vi "PI Controller with Stability Checker and Rate Limiter.vi"(2 "PI Parameters":T2, 3 "Tolerances":dbl[](array[numeric]), 4 "Feedback":dbl[](array[numeric]), 5 "CtrlIndex":i32, 7 "CommandCluster":T4, 9 "CmdLimits":cluster{"Step":dbl, "Max":dbl, "Min":dbl}, 10 "Rate Limits":T1={"Distant Rate"=50.0, "Close Rate"=0.5, "Error Cutoff"=10.0}, 11 "Stability In":T3, 12 "Controller?":bool, 13 "FF Scales":dbl[][](array[numeric])=[[0.0, 0.0, 0.0]]) -> (6 "Output":dbl, 8 "PIdata":dbl[](array[numeric]), 14 "Stable?":bool, 15 "Stability Out":T3)   [LabVIEW 2013]
uses:
  TypeDef/Command Cluster.ctl
  TypeDef/PI Parameters.ctl
  <vilib>/addons/control/pid/pid.llb/PID Output Rate Limiter (DBL).vi
  <vilib>/addons/control/pid/NI_PID_pid.lvlib
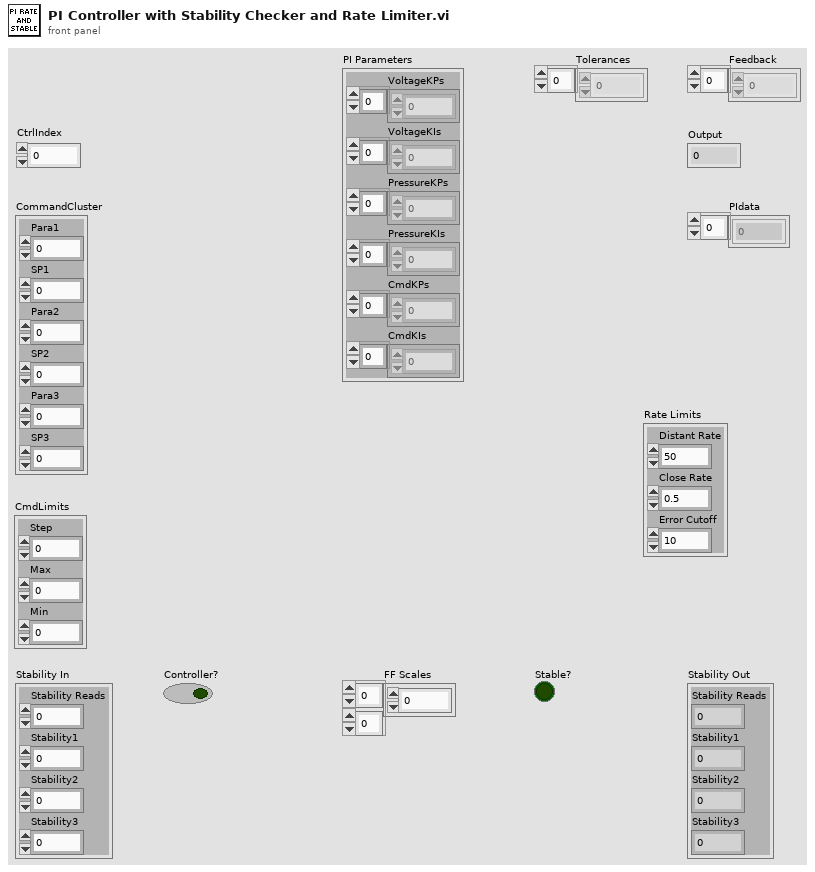
[diagram p1: front panel]
types:
  T1 = cluster{"Distant Rate":dbl, "Close Rate":dbl, "Error Cutoff":dbl}
  T2 = typedef "PI Parameters.ctl" = cluster{"VoltageKPs":dbl[], "VoltageKIs":dbl[], "PressureKPs":dbl[], "PressureKIs":dbl[], "CmdKPs":dbl[], "CmdKIs":dbl[]}
  T3 = cluster{"Stability Reads":i32, "Stability1":i32, "Stability2":i32, "Stability3":i32}
  T4 = typedef "Command Cluster.ctl" = cluster{"Para1":i32, "SP1":dbl, "Para2":i32, "SP2":dbl, "Para3":i32, "SP3":dbl}
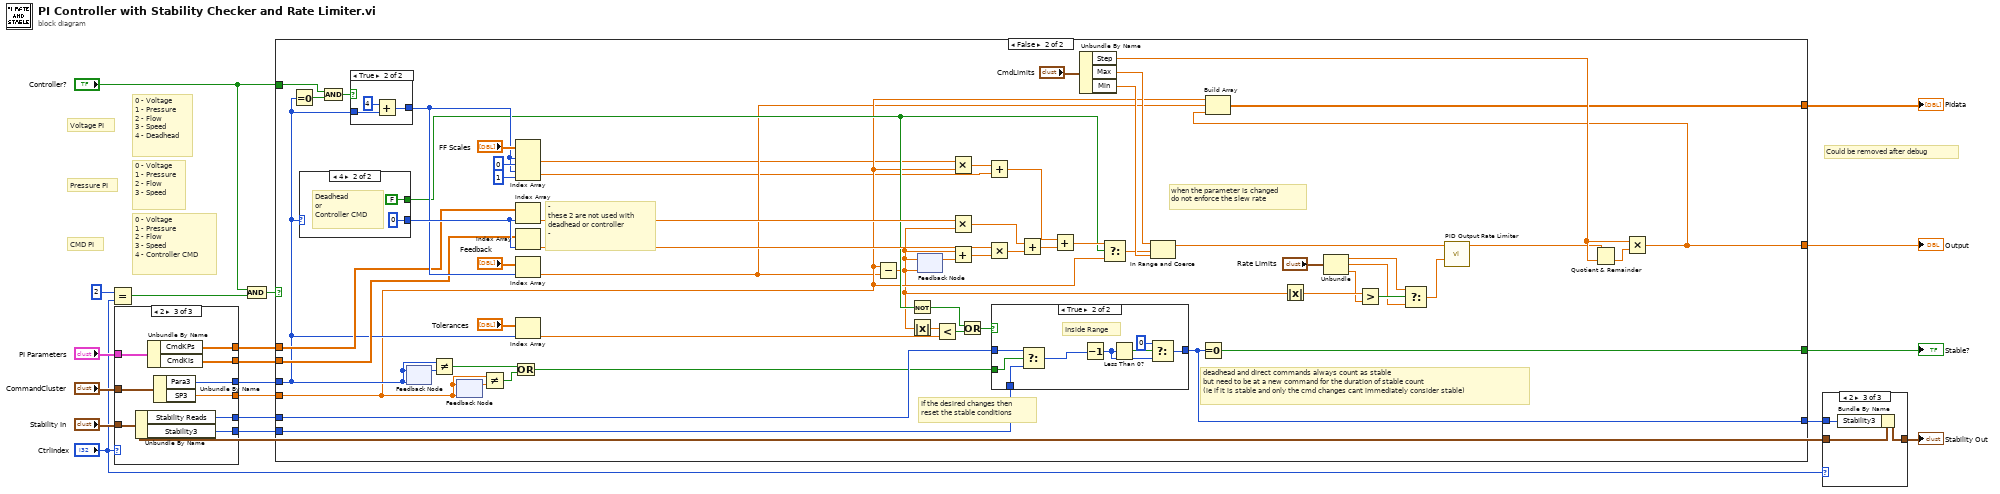
[diagram p0: block diagram]
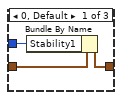
[diagram p2: hidden frame]
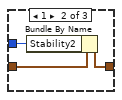
[diagram p3: hidden frame]
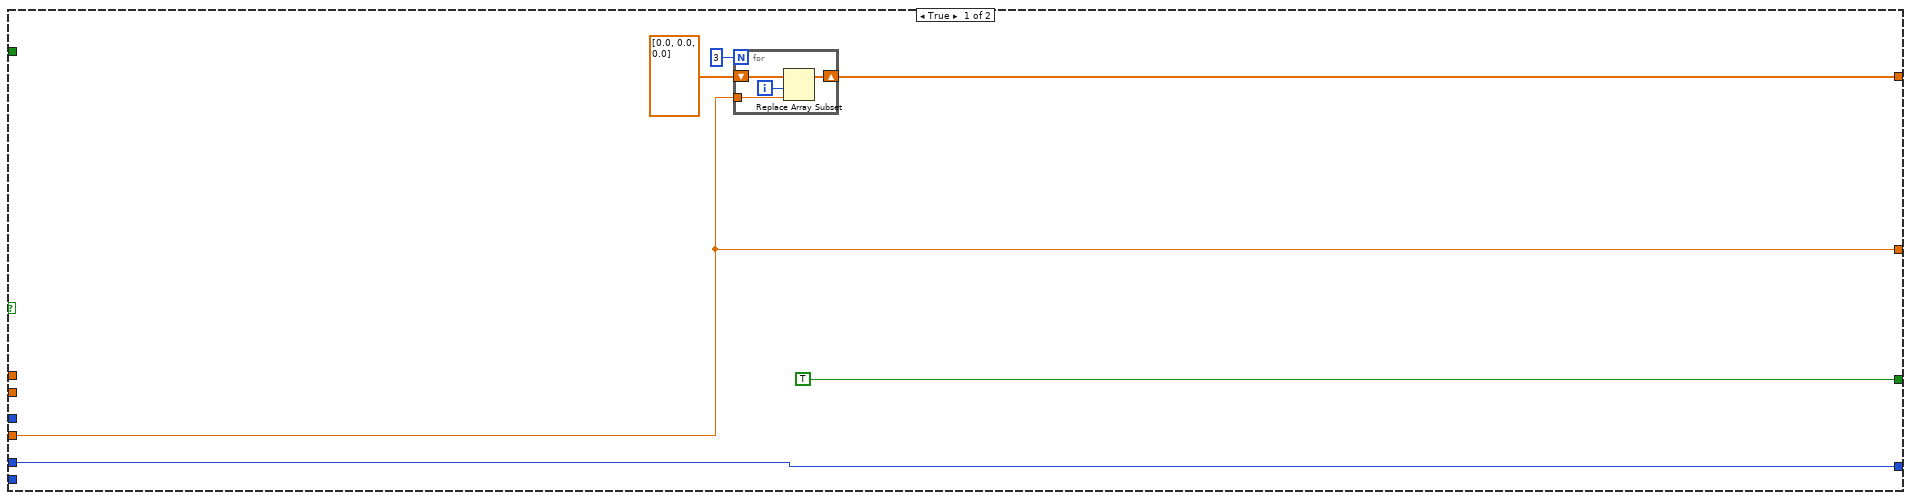
[diagram p4: hidden frame]
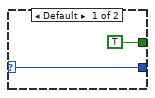
[diagram p7: hidden frame]
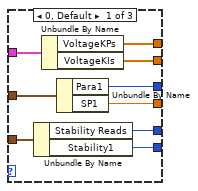
[diagram p8: hidden frame]
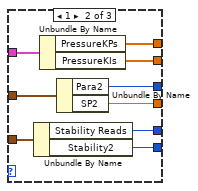
[diagram p9: hidden frame]
diagram:
  # "Could be removed after debug"
  # "CMD PI"
  # "Pressure PI"
  # "Voltage PI"
  # "0 - Voltage\n1 - Pressure\n2 - Flow\n3 - Speed\n4 - Controller CMD"
  # "0 - Voltage\n1 - Pressure\n2 - Flow\n3 - Speed"
  # "0 - Voltage\n1 - Pressure\n2 - Flow\n3 - Speed\n4 - Deadhead"
  n1 = Equal?(x=2, y="CtrlIndex") -> (x = y?=w10:bool)
  n2 = case shown="2" "CtrlIndex" {
    tunnel: "Stability In" -> [w28 w37 w46]
    tunnel: [w26 w35 w44] -> w18
    tunnel: [w27 w36 w45] -> w17
    tunnel: "CommandCluster" -> [w25 w34 w43]
    tunnel: [w24 w33 w42] -> w13
    tunnel: [w23 w32 w41] -> w12
    tunnel: "PI Parameters" -> [w22 w29 w40]
    tunnel: [w21 w31 w39] -> w14
    tunnel: [w20 w30 w38] -> w15
    frame 0, Default {
      n3 = Unbundle By Name(w28) -> ("Stability Reads"=w26:i32, "Stability1"=w27:i32)
      n4 = Unbundle By Name(w22) -> ("VoltageKPs"=w21:dbl[], "VoltageKIs"=w20:dbl[])
      n5 = Unbundle By Name(w25) -> ("Para1"=w24:i32, "SP1"=w23:dbl)
    }
    frame 1 {
      n6 = Unbundle By Name(w37) -> ("Stability Reads"=w35:i32, "Stability2"=w36:i32)
      n7 = Unbundle By Name(w29) -> ("PressureKPs"=w31:dbl[], "PressureKIs"=w30:dbl[])
      n8 = Unbundle By Name(w34) -> ("Para2"=w33:i32, "SP2"=w32:dbl)
    }
    frame 2 {
      n9 = Unbundle By Name(w46) -> ("Stability Reads"=w44:i32, "Stability3"=w45:i32)
      n10 = Unbundle By Name(w40) -> ("CmdKPs"=w39:dbl[], "CmdKIs"=w38:dbl[])
      n11 = Unbundle By Name(w43) -> ("Para3"=w42:i32, "SP3"=w41:dbl)
    }
  }
  n12 = And(x="Controller?", y=w10) -> (x .and. y?=w8:bool)
  n13 = case shown="False" w8 {
    tunnel: w18 -> [w51 w96]
    tunnel: w17 -> [_ w95]
    tunnel: w15 -> [_ w94]
    tunnel: w14 -> [_ w93]
    tunnel: w13 -> [_ w85]
    tunnel: w12 -> [w50 w74]
    tunnel: "Controller?" -> [_ w79]
    tunnel: [TRUE w78] -> w6
    tunnel: [w50 w58] -> w5
    tunnel: [w48 w77] -> w4
    tunnel: [w51 w76] -> w3
    frame True {
      n14 = for {
        N: 3 -> [_]
        shift-right: [w55] -> w48
        shift-left: dbl[] [0.0, 0.0, 0.0] -> [w56]
        tunnel: w50 -> [w53]
        i -> [w54]
        n15 = Replace Array Subset(array=w56, new element=w53, index=w54) -> (w55:dbl[])
      }
    }
    frame False {
      # "-\nthese 2 are not used with\ndeadhead or controller\n-"
      # "deadhead and direct commands always count as stable\nbut need to be at a new command for the duration of stable count\n(ie if it is stable and only the cmd changes cant immediately consider stable)"
      # "when the parameter is changed\ndo not enforce the slew rate"
      # "If the desired changes then\nreset the stable conditions"
      n16 = Equal To 0?(x=w85) -> (x = 0?=w101:bool)
      n17 = case shown="4" w85 {
        selector: w85 -> [w130 _]
        tunnel: [w130 0 ("index")] -> w99
        tunnel: [TRUE FALSE] -> w83
        frame Default {
        }
        frame 4 {
          # "Deadhead\nor\nController CMD"
        }
      }
      n18 = And(x=w79, y=w101) -> (x .and. y?=w100:bool)
      n19 = case shown="True" w100 {
        tunnel: w85 -> [w117 w120]
        tunnel: [w117 w118] -> w97
        frame False {
        }
        frame True {
          n20 = Add(x=4, y=w120) -> (x+y=w118:i32)
        }
      }
      n21 = feedback #1(w85) -> (w87:i32)
      n22 = feedback-in #1(w85) -> ()
      n23 = Not Equal?(x=w85, y=w87) -> (x != y?=w73:bool)
      n24 = feedback #2(w74) -> (w86:dbl)
      n25 = feedback-in #2(w74) -> ()
      n26 = Not Equal?(x=w74, y=w86) -> (x != y?=w71:bool)
      n27 = Or(x=w73, y=w71) -> (x .or. y?=w84:bool)
      n28 = Index Array(array="FF Scales", index (row) #1=w97, index (col) #1=0 ("disabled index (col)"), index (row) #2=w97, index (col) #2=1 ("disabled index (col)")) -> (element #1=w61:dbl, element #2=w60:dbl)
      n29 = Index Array(array=w93, index=w99) -> (element=w113:dbl)
      n30 = Index Array(array=w94, index=w99) -> (element=w111:dbl)
      n31 = Index Array(array="Feedback", index=w97) -> (element=w72:dbl)
      n32 = Index Array(array="Tolerances", index=w85) -> (element=w114:dbl)
      n33 = Subtract(x=w74, y=w72) -> (x-y=w69:dbl)
      n34 = Not(x=w83) -> (.not. x?=w82:bool)
      n35 = Absolute Value(x=w69) -> (abs(x)=w115:dbl)
      n36 = feedback #3(w69) -> (w108:dbl)
      n37 = feedback-in #3(w69) -> ()
      n38 = Less?(x=w115, y=w114) -> (x < y?=w81:bool)
      n39 = Multiply(x=w61, y=w74) -> (x*y=w62:dbl)
      n40 = Multiply(x=w113, y=w69) -> (x*y=w112:dbl)
      n41 = Add(x=w69, y=w108) -> (x+y=w109:dbl)
      n42 = Or(x=w82, y=w81) -> (x .or. y?=w80:bool)
      n43 = Add(x=w62, y=w60) -> (x+y=w103:dbl)
      n44 = Multiply(x=w111, y=w109) -> (x*y=w110:dbl)
      n45 = case shown="True" w80 {
        tunnel: [w121 w126] -> w76
        tunnel: w96 -> [w121 w124]
        tunnel: w95 -> [_ w123]
        tunnel: w84 -> [_ w125]
        frame False {
          # "Outside Range"
        }
        frame True {
          # "Inside Range"
          n46 = Select(t=w124, s=w125, f=w123) -> (s? t:f=w122:i32)
          n47 = Decrement(x=w122) -> (x-1=w128:i32)
          n48 = Less Than 0?(x=w128) -> (x < 0?=w127:bool)
          n49 = Select(t=0, s=w127, f=w128) -> (s? t:f=w126:i32)
        }
      }
      n50 = Add(x=w112, y=w110) -> (x+y=w106:dbl)
      n51 = Add(x=w103, y=w106) -> (x+y=w102:dbl)
      n52 = Unbundle By Name("CmdLimits") -> ("Step"=w89:dbl, "Max"=w90:dbl, "Min"=w91:dbl)
      n53 = Select(t=w102, s=w83, f=w74) -> (s? t:f=w75:dbl)
      n54 = In Range and Coerce(upper limit=w90, x=w75, lower limit=w91) -> (coerced(x)=w59:dbl)  [unwired: 1 out]
      n55 = Equal To 0?(x=w76) -> (x = 0?=w78:bool)
      n56 = Absolute Value(x=w69) -> (abs(x)=w68:dbl)
      n57 = Unbundle("Rate Limits") -> ("Distant Rate"=w65:dbl, "Close Rate"=w64:dbl, "Error Cutoff"=w67:dbl)
      n58 = Greater?(x=w68, y=w67) -> (0:w66:bool)
      n59 = Select(t=w65, s=w66, f=w64) -> (s? t:f=w63:dbl)
      n60 = call-poly <vilib>:"PID Output Rate Limiter.vi"("output rate (EGU/min)"=w63, "input (controller output)"=w59) -> ("output"=w57:dbl)  [unwired: 6 in, 1 out]
      n61 = Quotient & Remainder(x=w57, y=w89) -> (floor(x/y)=w88:dbl)  [unwired: 1 out]
      n62 = Multiply(x=w89, y=w88) -> (x*y=w58:dbl)
      n63 = Build Array(w74, w72, w58) -> (w77:dbl[])
    }
  }
  "Stable?" <- w6
  "Output" <- w5
  "PIdata" <- w4
  n64 = case shown="2" "CtrlIndex" {
    tunnel: "Stability In" -> [w135 w138 w141]
    tunnel: [w134 w137 w140] -> w7
    tunnel: w3 -> [w136 w139 w142]
    frame 0, Default {
      n65 = Bundle By Name(cluster=w135, "Stability1"=w136) -> (w134:T3)
    }
    frame 1 {
      n66 = Bundle By Name(cluster=w138, "Stability2"=w139) -> (w137:T3)
    }
    frame 2 {
      n67 = Bundle By Name(cluster=w141, "Stability3"=w142) -> (w140:T3)
    }
  }
  "Stability Out" <- w7
